vi "get voltage range byte.vi"(8 "error in (no error)":errorcluster caption="에러 입력(에러 없음)", 10 "voltage range":dbl, 11 "Haptic IC 입력":refnum<class "Haptic IC.lvclass">) -> (0 "error out":errorcluster caption="에러 출력", 2 "byte value":u8 format="%02x", 3 "Haptic IC 출력":refnum<class "Haptic IC.lvclass">)   [LabVIEW 2020, in "Haptic IC.lvclass"]
uses:
  Haptic IC.lvclass
  596c81d8-2ee9-4c9a-b356-8b1c4457a704.vi
  <vilib>/Comparison/Equal/Equal Functor/Equal Functor.lvclass
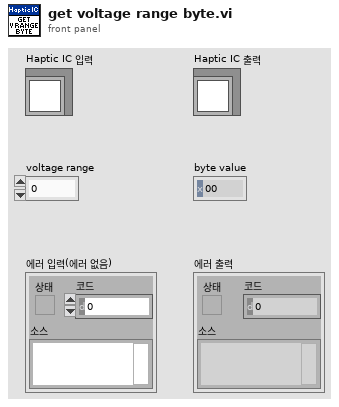
[diagram p1: front panel]
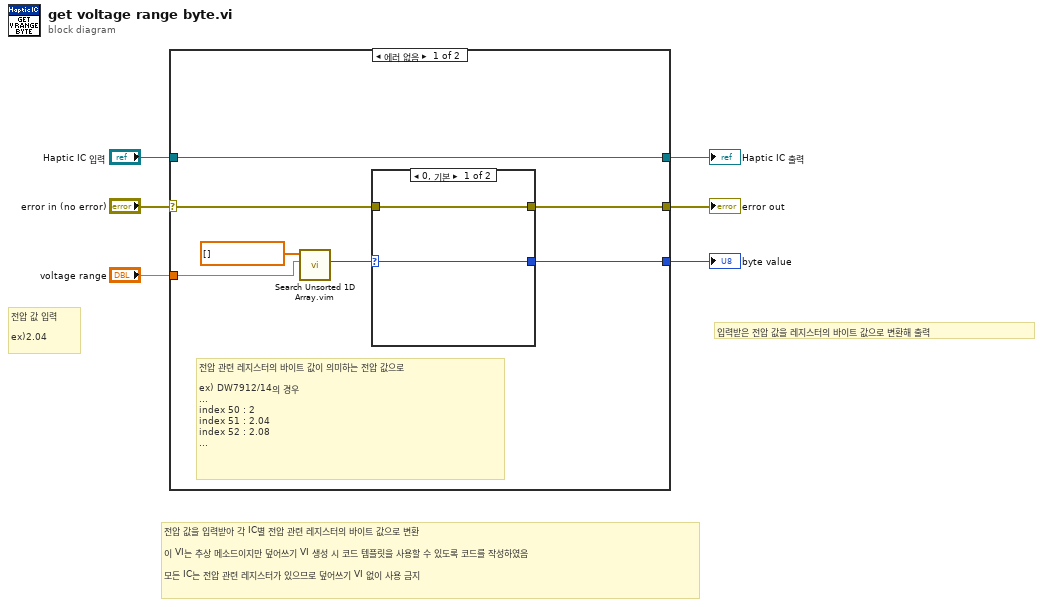
[diagram p0: block diagram]
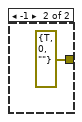
[diagram p2: hidden frame]
diagram:
  # "입력받은 전압 값을 레지스터의 바이트 값으로 변환해 출력"
  # "전압 값 입력\n\nex)2.04"
  # "전압 값을 입력받아 각 IC별 전압 관련 레지스터의 바이트 값으로 변환\n\n이 VI는 추상 메소드이지만 덮어쓰기 VI 생성 시 코드 템플릿을 사용할 수 있도록 코드를 작성하였음\n\n모든 IC는 전압 관련 레지스터가 있으므로 덮어쓰기 VI 없이 사용 금지"
  n1 = case shown="에러 없음" "error in (no error)" {
    selector: "error in (no error)" -> [w10 w18]
    tunnel: [w7 w18] -> w3
    tunnel: "Haptic IC 입력" -> [w13 w17]
    tunnel: [w13 w17] -> w5
    tunnel: "voltage range" -> [w11 _]
    tunnel: [w8 _] -> w1
    frame No Error {
      # "전압 관련 레지스터의 바이트 값이 의미하는 전압 값으로\n\nex) DW7912/14의 경우\n...\nindex 50 : 2\nindex 51 : 2.04\nindex 52 : 2.08\n..."
      n2 = call "Search Unsorted 1D Array.vim"("element"=w11, "unsorted 1D array"=dbl[] []) -> ("index of element"=w9:i32)  [unwired: 9 in]
      n3 = case shown="0, 기본" w9 {
        selector: w9 -> [w15 _]
        tunnel: w10 -> [w14 _]
        tunnel: [w15 _] -> w8
        tunnel: [w14 errorcluster {"status"=TRUE, "code"=0, "source"=""} ("error IO")] -> w7
        frame 0, Default {
        }
        frame -1 {
        }
      }
    }
    frame Error {
    }
  }
  "error out" <- w3
  "Haptic IC 출력" <- w5
  "byte value" <- w1
